vi "svc_Conditional Merge Error.vi"(7 "merge":bool, 10 "new error":errorcluster, 11 "error in (no error)":errorcluster) -> (3 "error out":errorcluster)   [LabVIEW 2017]
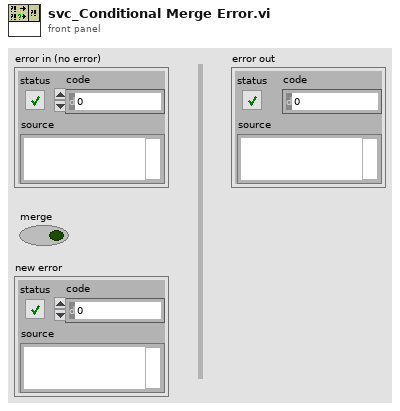
[diagram p1: front panel]
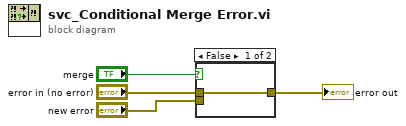
[diagram p0: block diagram]
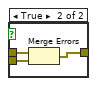
[diagram p2: hidden frame]
diagram:
  n1 = case shown="False" "merge" {
    tunnel: "new error" -> [_ w8]
    tunnel: [w5 w7] -> w2
    tunnel: "error in (no error)" -> [w5 w6]
    frame False {
    }
    frame True {
      n2 = Merge Errors(w6, w8) -> (w7:errorcluster)
    }
  }
  "error out" <- w2
